vi "Example Simple.vi"() -> ()   [LabVIEW 2013]
uses:
  C:/tf/play/labview/Tinkerforge.dll
  Tinkerforge.dll
panel:
  out "iaqIndexAccuracy":u8
  out "iaqIndex":i32
  out "airPressure (mbar)":sgl
  out "humidity (%RH)":sgl
  out "temperature (°C)":sgl
  in  "uid":string="abc"
  in  "port":i32=4223
  in  "host":string="localhost"
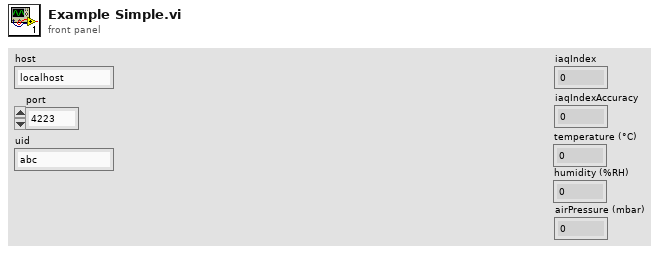
[diagram p1: front panel]
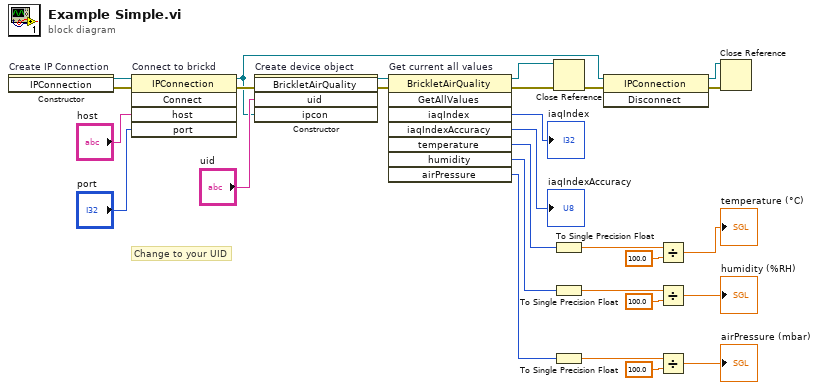
[diagram p0: block diagram]
diagram:
  # "Change to your UID"
  n1 = constructor on="Create IP Connection" class="IPConnection"() -> (reference out=w28:refnum<k24>, error out=w15:errorcluster)  [unwired: 3 in, 1 out]
  n2 = invoke on="Connect to brickd" class="IPConnection" method="Connect"(reference=w28, error in=w15, "host"="host", "port"="port") -> (reference out=w17:refnum<k24>, error out=w24:errorcluster)  [unwired: 1 in, 3 out]
  n3 = constructor on="Create device object" class="BrickletAirQuality"(error in=w24, "uid"="uid", "ipcon"=w17) -> (reference out=w22:refnum<k24>, error out=w23:errorcluster)  [unwired: 2 in, 3 out]
  n4 = invoke on="Get current all values" class="BrickletAirQuality" method="GetAllValues"(reference=w22, error in=w23) -> (reference out=w20:refnum<k24>, error out=w21:errorcluster, "iaqIndex"=→"iaqIndex":i32, "iaqIndexAccuracy"=→"iaqIndexAccuracy":u8, "temperature"=w5:i32, "humidity"=w4:i32, "airPressure"=w3:i32)  [unwired: 6 in, 1 out]
  n5 = Close Reference(reference=w20, error in (no error)=w21) -> (error out=w19:errorcluster)
  n6 = To Single Precision Float(number=w5) -> (single precision float=w13:sgl)
  n7 = To Single Precision Float(number=w4) -> (single precision float=w10:sgl)
  n8 = To Single Precision Float(number=w3) -> (single precision float=w8:sgl)
  n9 = invoke class="IPConnection" method="Disconnect"(reference=w17, error in=w19) -> (reference out=w16:refnum<k24>, error out=w18:errorcluster)  [unwired: 1 in, 1 out]
  n10 = Divide(x=w13, y=sgl 100.0) -> (x/y=→"temperature (°C)":sgl)
  n11 = Divide(x=w10, y=sgl 100.0) -> (x/y=→"humidity (%RH)":sgl)
  n12 = Divide(x=w8, y=sgl 100.0) -> (x/y=→"airPressure (mbar)":sgl)
  n13 = Close Reference(reference=w16, error in (no error)=w18) -> ()  [unwired: 1 out]
